vi "Eurotherm - Set P Term.vi"(0 "Eurotherm Setup In":T1={"Communication"={"Com Port"=1, "Address"=1, "Baud Rate"=9600}, "Name"="", "Enable"=FALSE, "Max Set Point"=0.0, "Min Set Point"=0.0, "Units"="", "Graph Data"=0, "Sensor type"=enum."RhFe", "Calibration File Path"=path "", "Conversion Type"=enum."Linear"} {"Min Set Point" format="%.3f"; "Max Set Point" format="%.3f"; "Communication"."Baud Rate" items=["300"=300, "600"=600, "1200"=1200, "2400"=2400, "4800"=4800, "9600 (default)"=9600, "19200"=19200, "38400"=38400, "57600"=57600, "76800"=76800, "115200"=115200, "230400"=230400]; "Communication"."Com Port" min=1 max=255; "Communication"."Address" min=1 max=99}, 7 "P Term":dbl=1.0 min=0.01 max=99.99 format="%.3f", 11 "error in (no error)":errorcluster) -> (4 "Eurotherm Setup Out":T1={"Communication"={"Com Port"=1, "Address"=1, "Baud Rate"=9600}, "Name"="", "Enable"=FALSE, "Max Set Point"=0.0, "Min Set Point"=0.0, "Units"="", "Graph Data"=0, "Sensor type"=enum."RhFe", "Calibration File Path"=path "", "Conversion Type"=enum."Linear"} {"Min Set Point" format="%.3f"; "Max Set Point" format="%.3f"; "Communication"."Baud Rate" items=["300"=300, "600"=600, "1200"=1200, "2400"=2400, "4800"=4800, "9600 (default)"=9600, "19200"=19200, "38400"=38400, "57600"=57600, "76800"=76800, "115200"=115200, "230400"=230400]; "Communication"."Com Port" min=1 max=255; "Communication"."Address" min=1 max=99}, 15 "error out":errorcluster)   [LabVIEW 2011]
uses:
  Eurotherm - Controls/Eurotherm - Setup.ctl
  Eurotherm - Controls/Eurotherm - Communication.ctl
  Common/Utilities/Controls - Com Ports/Com Port - Numeric.ctl
  Eurotherm - Controls/Eurotherm - Address.ctl
  Common/Utilities/Controls - Com Ports/Com Port - Baud Rate.ctl
  Common/Utilities - System/Sensors/Sensors - Controls/Sensors - Temperature Sensor Type.ctl
  Common/Utilities - System/Sensors/Sensors - Controls/Sensors - Conversion Type.ctl
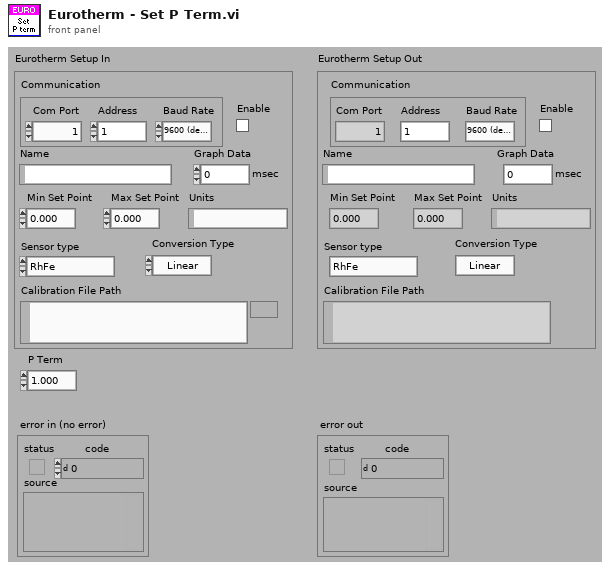
[diagram p1: front panel]
types:
  T1 = typedef "Eurotherm - Setup.ctl" = cluster{"Communication":T2, "Name":string, "Enable":bool, "Max Set Point":dbl, "Min Set Point":dbl, "Units":string, "Graph Data":u32, "Sensor type":T6, "Calibration File Path":path, "Conversion Type":T7}
  T2 = typedef "Eurotherm - Communication.ctl" = cluster{"Com Port":T3, "Address":T4, "Baud Rate":T5}
  T3 = typedef "Com Port - Numeric.ctl" = i32
  T4 = typedef "Eurotherm - Address.ctl" = u8
  T5 = typedef "Com Port - Baud Rate.ctl" = u32
  T6 = typedef "Sensors - Temperature Sensor Type.ctl" = enum16{"RhFe", "Pt", "K type thermocouple", "W5 type thermocouple", "No Conversion"}
  T7 = typedef "Sensors - Conversion Type.ctl" = enum16{"Linear", "Spline"}
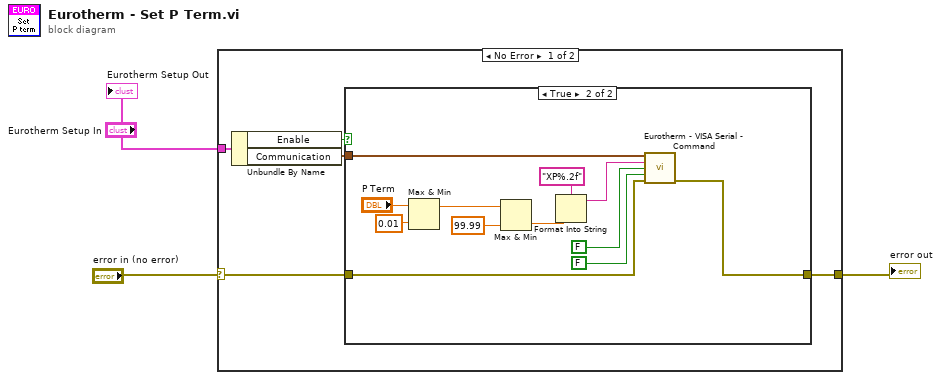
[diagram p0: block diagram]
diagram:
  n1 = case shown="No Error" "error in (no error)" {
    selector: "error in (no error)" -> [w8 w22]
    tunnel: [w7 w22] -> w2
    tunnel: "Eurotherm Setup In" -> [w4 _]
    frame No Error {
      n2 = Unbundle By Name(w4) -> ("Enable"=w5:bool, "Communication"=w6:T2)
      n3 = case shown="True" w5 {
        tunnel: w8 -> [w9 w15]
        tunnel: [w9 w18] -> w7
        tunnel: w6 -> [_ w19]
        frame False {
        }
        frame True {
          n4 = Max & Min(x="P Term", y=0.01) -> (max(x,y)=w13:dbl)  [unwired: 1 out]
          n5 = Max & Min(x=w13, y=99.99) -> (min(x,y)=w12:dbl)  [unwired: 1 out]
          n6 = Format Into String(format string="XP%.2f", w12) -> (resulting string=w16:string)  [unwired: 2 in, 1 out]
          n7 = call "Eurotherm - VISA Serial - Command.vi"("VISA resource name In (String)"=w19, "Command"=w16, "Read Reply"=FALSE, "Close Session"=FALSE, "error in (no error)"=w15) -> ("error out"=w18:errorcluster)  [unwired: 8 in, 2 out]
        }
      }
    }
    frame Error {
    }
  }
  "error out" <- w2
  "Eurotherm Setup Out" <- "Eurotherm Setup In"
